vi "Save Folder Config.vi"(7 "Folder Config":T1[](array[typedef]), 8 "error in (no error)":errorcluster, 10 "Name":string, 11 "INI Filename":string) -> (0 "error out":errorcluster)   [LabVIEW 2020, in "Negentropic IDE.lvlib"]
uses:
  Negentropic IDE.lvlib
  Folder Config.ctl
  Scope.ctl
  <vilib>/Utility/config.llb/Write Key (String).vi
  <vilib>/Utility/config.llb/NI_LVConfig.lvlib
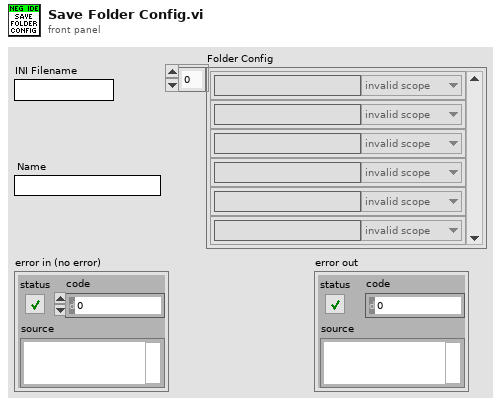
[diagram p1: front panel]
types:
  T1 = typedef "Negentropic IDE.lvlib/Folder Config.ctl" = cluster{"Path":string, "Scope":T2}
  T2 = typedef "Negentropic IDE.lvlib/Scope.ctl" = enum32{"invalid scope", "public", "private", "protected", "community"}
  T3 = typedef "NI_LVConfig.lvlib/Config Data RefNum.ctl" = refnum<k1>
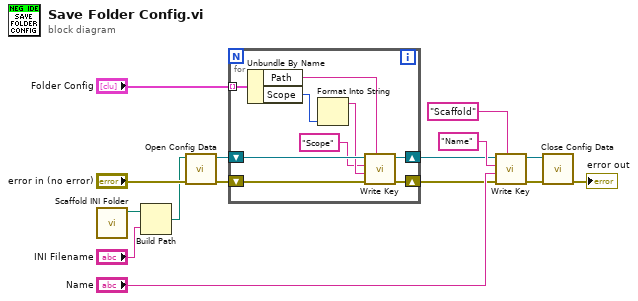
[diagram p0: block diagram]
diagram:
  n1 = call "Scaffold INI Folder.vi"() -> ("Scaffold INI Folder"=w9:path)  [unwired: 10 in, 1 out]
  n2 = Build Path(base path=w9, name or relative path="INI Filename") -> (appended path=w11:path)
  n3 = call <vilib>:"Open Config Data.vi"("error in (no error)"="error in (no error)", "configuration file path"=w11) -> ("error out"=w2:errorcluster, "refnum"=w3:T3)  [unwired: 7 in, 1 out]
  n4 = for {
    tunnel: "Folder Config" -> [w24] mode=indexing
    shift-right: [w16] -> w6
    shift-left: w2 -> [w22]
    shift-right: [w17] -> w5
    shift-left: w3 -> [w23]
    n5 = Unbundle By Name(w24) -> ("Path"=w21:string, "Scope"=w20:T2)
    n6 = Format Into String(w20) -> (resulting string=w19:string)  [unwired: 3 in, 1 out]
    n7 = call-poly <vilib>:"Write Key.vi"("section"=w21, "error in (no error)"=w22, "value"=w19, "key"="Scope", "refnum"=w23) -> ("error out"=w16:errorcluster, "refnum out"=w17:T3)  [unwired: 4 in, 1 out]
  }
  n8 = call-poly <vilib>:"Write Key.vi"("section"="Scaffold", "error in (no error)"=w6, "value"="Name", "key"="Name", "refnum"=w5) -> ("error out"=w15:errorcluster, "refnum out"=w14:T3)  [unwired: 4 in, 1 out]
  n9 = call <vilib>:"Close Config Data.vi"("error in (no error)"=w15, "refnum"=w14) -> ("error out"=→"error out":errorcluster)  [unwired: 8 in, 1 out]
